vi "Sequencer Main.vi"() -> ()   [LabVIEW 2018] (continued)
                              # "Calculate Values"
                              n2034 = local read "Channel A"() -> (w4088:cluster{i32, dbl, dbl[]})
                              n2035 = local read "Channel B"() -> (w4085:cluster{i32, dbl, dbl[]})
                              n2036 = Unbundle(w4088) -> (w4093:dbl[])  [unwired: 2 out]
                              n2037 = Unbundle(w4085) -> (w4097:dbl[])  [unwired: 2 out]
                              n2038 = Array Size(array=w4093) -> (size(s)=w4099:i32)
                              n2039 = Array Size(array=w4097) -> (size(s)=w4096:i32)
                              n2040 = Subtract(x=w4099, y=w4095) -> (x-y=w4098:i32)
                              n2041 = Array Subset(array=w4093, index=w4095, length=w4098) -> (w4076:dbl[])
                              n2042 = Add(x=290, y="Correction") -> (x+y=w4077:i32)
                              "Pico Scope Correction" <- w4077
                              n2043 = Subtract(x=w4096, y=w4095) -> (x-y=w4094:i32)
                              n2044 = Array Subset(array=w4097, index=w4095, length=w4094) -> (w4090:dbl[])
                              n2045 = call "Wave Filter.vi"("Filter ON"=w4064, "Value"="F-Value", "Data In"=w4076) -> ("Data Out"=w4086:dbl[])  [unwired: 8 in]
                              n2046 = call "Wave Filter.vi"("Filter ON"=w4064, "Value"="F-Value", "Data In"=w4090) -> ("Data Out"=w4081:dbl[])  [unwired: 8 in]
                              n2047 = call "Convert to Dynamic Data"("Array"=w4086) -> ("Dynamic Data Type"=w4073:dynamicdata)  [unwired: 3 in]
                              n2048 = call "Convert to Dynamic Data2"("Array"=w4081) -> ("Dynamic Data Type"=w4072:dynamicdata)  [unwired: 3 in]
                              n2049 = Bundle(cluster=w4085, w4081) -> (w4084:cluster{i32, dbl, dbl[]})  [unwired: 2 in]
                              n2050 = call "Amplitude and Level Measurements2"("Signals"=w4072) -> ("Mean (DC)"=w4074:dynamicdata, "Negative Peak"=w4079:dynamicdata, "Positive Peak"=w4080:dynamicdata, "Peak to Peak"=w4070:dynamicdata)  [unwired: 10 in, 1 out]
                              n2051 = Bundle(cluster=w4088, w4086) -> (w4087:cluster{i32, dbl, dbl[]})  [unwired: 2 in]
                              n2052 = call "Amplitude and Level Measurements"("Signals"=w4073) -> ("Mean (DC)"=w4075:dynamicdata, "Negative Peak"=w4082:dynamicdata, "Positive Peak"=w4083:dynamicdata, "Peak to Peak"=w4067:dynamicdata)  [unwired: 10 in, 1 out]
                              n2053 = local write "Channel B"(w4084) -> ()
                              n2054 = Divide(x=w4067, y=2.0) -> (x/y=w4066:dynamicdata)
                              n2055 = Divide(x=w4070, y=2.0) -> (x/y=w4069:dynamicdata)
                              n2056 = local write "Channel A"(w4087) -> ()
                              n2057 = Subtract(1:w4075, 2:w4083) -> (0:w4109:dynamicdata)  [unwired: 1 in, 1 out]
                              n2058 = Add(1:w4075, 2:w4082) -> (0:w4108:dynamicdata)  [unwired: 1 in, 1 out]
                              n2059 = Subtract(1:w4074, 2:w4080) -> (0:w4105:dynamicdata)  [unwired: 1 in, 1 out]
                              n2060 = Add(1:w4074, 2:w4079) -> (0:w4104:dynamicdata)  [unwired: 1 in, 1 out]
                              n2061 = Multiply(x=w4066, y=w4077) -> (x*y=w4107:dynamicdata)
                              n2062 = Multiply(x=w4109, y=w4077) -> (x*y=w4103:dynamicdata)
                              n2063 = Multiply(x=w4108, y=w4077) -> (x*y=w4102:dynamicdata)
                              n2064 = local read "Measure Ch-A"() -> (w4113:T10)
                              n2065 = Multiply(x=w4069, y=w4077) -> (x*y=w4106:dynamicdata)
                              n2066 = Multiply(x=w4105, y=w4077) -> (x*y=w4101:dynamicdata)
                              n2067 = Multiply(x=w4104, y=w4077) -> (x*y=w4100:dynamicdata)
                              n2068 = Bundle By Name(cluster=w4113, "MAX Vpp"=w4103, "PickToPoick / 2"=w4107, "MIN Vpp"=w4102) -> (w4112:T10)
                              n2069 = local read "Measure Ch-B"() -> (w4110:T9)
                              n2070 = Bundle By Name(cluster=w4110, "MAX Vpp"=w4101, "PickToPick / 2"=w4106, "MIN Vpp"=w4100) -> (w4111:T9)
                              n2071 = local write "Measure Ch-B"(w4111) -> ()
                              n2072 = local write "Measure Ch-A"(w4112) -> ()
                            }
                            frame #2 {
                              # "GoTo Test-nmb"
                              # "ReTest Cyckles"
                              # "Select Channel & Set Retest Parametrs in FALSE Case"
                              n2073 = Index Array(array=w4131, index #1=0 ("index"), index #2=1 ("index"), index #3=2 ("index")) -> (element #1=w4135:string, element #2=w4136:string, element #3=w4137:string)
                              n2074 = global read "Global Variable.vi" "Retest Cnt"() -> (w4130:i16)
                              n2075 = local read "Debugging"() -> (w4128:bool)
                              n2076 = To Upper Case(1:w4135) -> (0:w4127:string)
                              n2077 = call "Convert from Dynamic Data"("Dynamic Data Type"=w4123) -> ("Scalar"=w4119:dbl)  [unwired: 3 in]
                              n2078 = call "Convert from Dynamic Data2"("Dynamic Data Type"=w4122) -> ("Scalar"=w4118:dbl)  [unwired: 3 in]
                              n2079 = call "Convert from Dynamic Data3"("Dynamic Data Type"=w4121) -> ("Scalar"=w4117:dbl)  [unwired: 3 in]
                              n2080 = call "Convert from Dynamic Data4"("Dynamic Data Type"=w4120) -> ("Scalar"=w4116:dbl)  [unwired: 3 in]
                              n2081 = Decimal String To Number(string=w4137) -> (number=w4124:i32)  [unwired: 2 in, 1 out]
                              n2082 = Decimal String To Number(string=w4136) -> (number=w4126:i32)  [unwired: 2 in, 1 out]
                              n2083 = Equal?(x=w4130, y=i16 0) -> (x = y?=w4125:bool)
                              n2084 = case shown="False" w4128 {
                                tunnel: w4127 -> [w4142 _]
                                tunnel: w4125 -> [w4139 _]
                                tunnel: w4124 -> [w4141 _]
                                tunnel: w4126 -> [w4140 _]
                                frame False {
                                n2085 = case shown="\"FALSE\"" w4142 {
                                tunnel: w4139 -> [_ w4146]
                                tunnel: w4141 -> [_ w4143]
                                tunnel: w4140 -> [_ w4144]
                                frame "Idle", Default {
                                }
                                frame "FALSE" {
                                n2086 = global write "Global Variable.vi" "Retest Step Nmb"(w4144) -> ()
                                n2087 = global write "Global Variable.vi" "Retest Nmb"(w4143) -> ()
                                n2088 = case shown="True" w4146 {
                                tunnel: w4143 -> [_ w4150]
                                tunnel: w4144 -> [_ _]
                                frame False {
                                n2089 = global read "Global Variable.vi" "Retest Cnt"() -> (w4148:i16)
                                n2090 = Decrement(x=w4148) -> (x-1=w4147:i16)
                                n2091 = global write "Global Variable.vi" "Retest Cnt"(w4147) -> ()
                                }
                                frame True {
                                # "if(Retest-OFF & Cnt=0)"
                                n2092 = Decrement(x=w4150) -> (x-1=w4149:i32)
                                n2093 = global write "Global Variable.vi" "Retest Cnt"(w4149) -> ()
                                }
                                }
                                n2094 = global write "Global Variable.vi" "Retest ON"(TRUE ("Retest ON")) -> ()
                                }
                                }
                                }
                                frame True {
                                }
                              }
                              n2095 = case shown="\"A\", Default" w4138 {
                                tunnel: [w4152 w4154] -> w4115
                                tunnel: w4119 -> [w4152 _]
                                tunnel: w4118 -> [w4151 _]
                                tunnel: [w4151 w4153] -> w4114
                                tunnel: w4117 -> [_ w4154]
                                tunnel: w4116 -> [_ w4153]
                                frame "A", Default {
                                }
                                frame "B" {
                                }
                              }
                            }
                            frame #3 {
                              # "Negative MIN"
                              # "Positive MAX"
                              n2096 = Multiply(x="Delay", y=u32 1000 ("milliseconds to wait")) -> (x*y=w4157:u32)
                              n2097 = Wait (ms)(milliseconds to wait=w4157) -> ()  [unwired: 1 out]
                            }
                          }
                          n2098 = in-place {
                            in-place-border: w3995 -> [w4019]
                            in-place-border: w3993 -> [w4018]
                            in-place-border: w3996 -> [w4025]
                            in-place-border: w3997 -> [w4024]
                            in-place-border: [w4026] -> w3991
                            in-place-border: [w4017] -> w3990
                            # "Step Result Msg"
                            # "Step TEST Result"
                            n2099 = in-place {
                              in-place-border: w4025 -> [w4030]
                              in-place-border: w4024 -> [w4027]
                              in-place-border: [w4030] -> w4023
                              in-place-border: [w4029] -> w4021
                              in-place-border: [w4028] -> w4020
                              in-place-border: [w4027] -> w4022
                              n2100 = Multiply(x=w4027, y=-1.0) -> (x*y=w4028:dbl)
                              n2101 = Multiply(x=w4030, y=-1.0) -> (x*y=w4029:dbl)
                            }
                            n2102 = In Range and Coerce(upper limit=w4023, x=w4019, lower limit=w4022) -> (In Range?=w4015:bool)  [unwired: 1 out]
                            n2103 = In Range and Coerce(upper limit=w4020, x=w4018, lower limit=w4021) -> (In Range?=w4014:bool)  [unwired: 1 out]
                            n2104 = And(x=w4015, y=w4014) -> (x .and. y?=w4013:bool)
                            n2105 = case shown="False" w4013 {
                              tunnel: [enum16{"Idle", "PASS", "FALSE"}."FALSE" ("Step Test Result") enum16{"Idle", "PASS", "FALSE"}."PASS" ("Step Test Result")] -> w4026
                              frame False {
                              }
                              frame True {
                              }
                            }
                            n2106 = Format Into String(format string="Max: %.1fVAC :: Min: %.1fVAC", w4019, w4018) -> (resulting string=w4017:string)  [unwired: 2 in, 1 out]
                          }
                        }
                        frame 56 {
                          # "Read Peack To Peak / 2"
                          # "Lover Lim"
                          # "Upper Lim"
                          # "PicoScope"
                          # "PicoScope Case"
                          n2107 = Unbundle By Name(w4178) -> ("Parameters"=w4172:string, "Test Values.Upper Limit"=w4176:dbl, "Test Values.Lower Limit"=w4175:dbl, "Test Values.Numeric Value"=w4177:dbl)
                          n2108 = property on="Tab Control Msg" class="TabCtl (strict)"("Value"=T21."Scope" ("Tab Control Msg")) -> (error out=w4174:errorcluster)  [unwired: 2 in, 1 out]
                          n2109 = flat-sequence {
                            tunnel: w4177 -> [w4205]
                            tunnel: w4176 -> [w4198]
                            tunnel: w4175 -> [w4197]
                            tunnel: w4174 -> [_]
                            tunnel: [w4198] -> w4164
                            tunnel: [w4197] -> w4165
                            tunnel: w4172 -> [w4196]
                            tunnel: [w4194] -> w4169
                            tunnel: [w4190] -> w4166
                            tunnel: [w4224] -> w4171
                            tunnel: [w4223] -> w4170
                            tunnel: w4169 -> [w4249]
                            tunnel: [w4249] -> w4168
                            tunnel: [w4248] -> w4167
                            tunnel: w4166 -> [w4248]
                            tunnel: w4171 -> [w4273]
                            tunnel: w4170 -> [w4272]
                            tunnel: w4168 -> [w4288]
                            tunnel: w4167 -> [w4281]
                            tunnel: [w4271] -> w4162
                            tunnel: [w4304] -> w4163
                            tunnel: w4162 -> [w4304]
                            frame #0 {
                              n2110 = while {
                                shift-right: [w4216] -> _
                                shift-left: w4196 -> [w4217]
                                tunnel: [w4213] -> w4195 mode=indexing
                                stop <- w4215 stop-if-true
                                # "Get Array of Parametrs"
                                n2111 = Match Pattern(string=w4217, regular expression=">") -> (before substring=w4213:string, after substring=w4216:string, offset past match=w4214:i32)  [unwired: 1 in, 1 out]
                                n2112 = Less Than 0?(x=w4214) -> (x < 0?=w4215:bool)
                              }
                              n2113 = Multiply(x=w4197, y=-0.2) -> (x*y=w4200:dbl)
                              n2114 = Bundle("Lower Limit"=w4197, "Upper Limit"=w4198, "Numeric Value"=w4205) -> (w4206:T36)  [unwired: 1 in]
                              n2115 = Multiply(x=w4198, y=0.2) -> (x*y=w4202:dbl)
                              n2116 = Add(x=w4200, y=w4197) -> (x+y=w4199:dbl)
                              n2117 = property on="Limits" class="Slide (strict)"("Value"=w4206) -> ()  [unwired: 2 in, 2 out]
                              n2118 = Add(x=w4202, y=w4198) -> (x+y=w4201:dbl)
                              n2119 = property on="Limits" class="Slide (strict)"("Scale.Maximum"=w4201, "Scale.Minimum"=w4199) -> ()  [unwired: 2 in, 2 out]
                              n2120 = Index Array(array=w4195, index #1=0 ("index"), index #2=1 ("index")) -> (element #1=w4194:string, element #2=w4191:string)
                              n2121 = while {
                                shift-right: [w4210] -> _
                                shift-left: w4191 -> [w4211]
                                tunnel: [w4207] -> w4190 mode=indexing
                                stop <- w4209 stop-if-true
                                # "Get Array of Sub Parametrs"
                                n2122 = Match Pattern(string=w4211, regular expression=":") -> (before substring=w4207:string, after substring=w4210:string, offset past match=w4208:i32)  [unwired: 1 in, 1 out]
                                n2123 = Less Than 0?(x=w4208) -> (x < 0?=w4209:bool)
                              }
                            }
                            frame #1 {
                              w4219 = TRUE
                              w4252 = 100 ("index")
                              # "700"
                              # "Devider compensite"
                              # "remove first\nxx element (noise)"
                              # "Ch-B Peack To Peack / 2"
                              # "Ch-A Peack To Peack / 2"
                              # "Res Devider Compens\n100K / 10K"
                              # "Calculate Values"
                              n2124 = local read "Correction"() -> (w4222:i32)
                              n2125 = local read "Channel A"() -> (w4246:cluster{i32, dbl, dbl[]})
                              n2126 = local read "Channel B"() -> (w4243:cluster{i32, dbl, dbl[]})
                              n2127 = Unbundle(w4246) -> (w4250:dbl[])  [unwired: 2 out]
                              n2128 = Unbundle(w4243) -> (w4254:dbl[])  [unwired: 2 out]
                              n2129 = local read "F-Value"() -> (w4220:dbl)
                              n2130 = Array Size(array=w4250) -> (size(s)=w4256:i32)
                              n2131 = Array Size(array=w4254) -> (size(s)=w4253:i32)
                              n2132 = Subtract(x=w4256, y=w4252) -> (x-y=w4255:i32)
                              n2133 = Array Subset(array=w4250, index=w4252, length=w4255) -> (w4235:dbl[])
                              n2134 = Add(x=290, y=w4222) -> (x+y=w4221:i32)
                              n2135 = Subtract(x=w4253, y=w4252) -> (x-y=w4251:i32)
                              n2136 = Array Subset(array=w4254, index=w4252, length=w4251) -> (w4247:dbl[])
                              n2137 = call "Wave Filter.vi"("Filter ON"=w4219, "Value"=w4220, "Data In"=w4235) -> ("Data Out"=w4244:dbl[])  [unwired: 8 in]
                              n2138 = call "Wave Filter.vi"("Filter ON"=w4219, "Value"=w4220, "Data In"=w4247) -> ("Data Out"=w4239:dbl[])  [unwired: 8 in]
                              n2139 = local write "Pico Scope Correction"(w4221) -> ()
                              n2140 = call "Convert to Dynamic Data4"("Array"=w4244) -> ("Dynamic Data Type"=w4232:dynamicdata)  [unwired: 3 in]
                              n2141 = call "Convert to Dynamic Data3"("Array"=w4239) -> ("Dynamic Data Type"=w4231:dynamicdata)  [unwired: 3 in]
                              n2142 = Bundle(cluster=w4243, w4239) -> (w4242:cluster{i32, dbl, dbl[]})  [unwired: 2 in]
                              n2143 = call "Amplitude and Level Measurements4"("Signals"=w4231) -> ("Mean (DC)"=w4233:dynamicdata, "Negative Peak"=w4237:dynamicdata, "Positive Peak"=w4238:dynamicdata, "Peak to Peak"=w4230:dynamicdata)  [unwired: 10 in, 1 out]
                              n2144 = Bundle(cluster=w4246, w4244) -> (w4245:cluster{i32, dbl, dbl[]})  [unwired: 2 in]
                              n2145 = call "Amplitude and Level Measurements3"("Signals"=w4232) -> ("Mean (DC)"=w4234:dynamicdata, "Negative Peak"=w4240:dynamicdata, "Positive Peak"=w4241:dynamicdata, "Peak to Peak"=w4227:dynamicdata)  [unwired: 10 in, 1 out]
                              n2146 = local write "Channel B"(w4242) -> ()
                              n2147 = Divide(x=w4227, y=2.0) -> (x/y=w4226:dynamicdata)
                              n2148 = Divide(x=w4230, y=2.0) -> (x/y=w4229:dynamicdata)
                              n2149 = local write "Channel A"(w4245) -> ()
                              n2150 = Subtract(1:w4234, 2:w4241) -> (0:w4264:dynamicdata)  [unwired: 1 in, 1 out]
                              n2151 = Add(1:w4234, 2:w4240) -> (0:w4263:dynamicdata)  [unwired: 1 in, 1 out]
                              n2152 = Subtract(1:w4233, 2:w4238) -> (0:w4262:dynamicdata)  [unwired: 1 in, 1 out]
                              n2153 = Add(1:w4233, 2:w4237) -> (0:w4261:dynamicdata)  [unwired: 1 in, 1 out]
                              n2154 = Multiply(x=w4226, y=w4221) -> (x*y=w4224:dynamicdata)
                              n2155 = Multiply(x=w4264, y=w4221) -> (x*y=w4260:dynamicdata)
                              n2156 = Multiply(x=w4263, y=w4221) -> (x*y=w4259:dynamicdata)
                              n2157 = local read "Measure Ch-A"() -> (w4268:T10)
                              n2158 = Multiply(x=w4229, y=w4221) -> (x*y=w4223:dynamicdata)
                              n2159 = Multiply(x=w4262, y=w4221) -> (x*y=w4258:dynamicdata)
                              n2160 = Multiply(x=w4261, y=w4221) -> (x*y=w4257:dynamicdata)
                              n2161 = Bundle By Name(cluster=w4268, "MAX Vpp"=w4260, "PickToPoick / 2"=w4224, "MIN Vpp"=w4259) -> (w4267:T10)
                              n2162 = local read "Measure Ch-B"() -> (w4265:T9)
                              n2163 = Bundle By Name(cluster=w4265, "MAX Vpp"=w4258, "PickToPick / 2"=w4223, "MIN Vpp"=w4257) -> (w4266:T9)
                              n2164 = local write "Measure Ch-B"(w4266) -> ()
                              n2165 = local write "Measure Ch-A"(w4267) -> ()
                            }
                            frame #2 {
                              # "GoTo Test-nmb"
                              # "ReTest Cyckles"
                              # "Select Channel & Set Retest Parametrs in FALSE Case"
                              n2166 = Index Array(array=w4281, index #1=0 ("index"), index #2=1 ("index"), index #3=2 ("index")) -> (element #1=w4285:string, element #2=w4286:string, element #3=w4287:string)
                              n2167 = global read "Global Variable.vi" "Retest Cnt"() -> (w4280:i16)
                              n2168 = local read "Debugging"() -> (w4278:bool)
                              n2169 = To Upper Case(1:w4285) -> (0:w4277:string)
                              n2170 = call "Convert from Dynamic Data8"("Dynamic Data Type"=w4273) -> ("Scalar"=w4269:dbl)  [unwired: 3 in]
                              n2171 = call "Convert from Dynamic Data6"("Dynamic Data Type"=w4272) -> ("Scalar"=w4270:dbl)  [unwired: 3 in]
                              n2172 = Decimal String To Number(string=w4287) -> (number=w4274:i32)  [unwired: 2 in, 1 out]
                              n2173 = Decimal String To Number(string=w4286) -> (number=w4276:i32)  [unwired: 2 in, 1 out]
                              n2174 = Equal?(x=w4280, y=i16 0) -> (x = y?=w4275:bool)
                              n2175 = case shown="False" w4278 {
                                tunnel: w4277 -> [w4292 _]
                                tunnel: w4275 -> [w4289 _]
                                tunnel: w4274 -> [w4291 _]
                                tunnel: w4276 -> [w4290 _]
                                frame False {
                                n2176 = case shown="\"FALSE\"" w4292 {
                                tunnel: w4289 -> [_ w4296]
                                tunnel: w4291 -> [_ w4293]
                                tunnel: w4290 -> [_ w4294]
                                frame "Idle", Default {
                                }
                                frame "FALSE" {
                                n2177 = global write "Global Variable.vi" "Retest Step Nmb"(w4294) -> ()
                                n2178 = global write "Global Variable.vi" "Retest Nmb"(w4293) -> ()
                                n2179 = case shown="True" w4296 {
                                tunnel: w4293 -> [_ w4300]
                                tunnel: w4294 -> [_ _]
                                frame False {
                                n2180 = global read "Global Variable.vi" "Retest Cnt"() -> (w4298:i16)
                                n2181 = Decrement(x=w4298) -> (x-1=w4297:i16)
                                n2182 = global write "Global Variable.vi" "Retest Cnt"(w4297) -> ()
                                }
                                frame True {
                                # "if(Retest-OFF & Cnt=0)"
                                n2183 = Decrement(x=w4300) -> (x-1=w4299:i32)
                                n2184 = global write "Global Variable.vi" "Retest Cnt"(w4299) -> ()
                                }
                                }
                                n2185 = global write "Global Variable.vi" "Retest ON"(TRUE ("Retest ON")) -> ()
                                }
                                }
                                }
                                frame True {
                                }
                              }
                              n2186 = case shown="\"A\", Default" w4288 {
                                tunnel: [w4301 w4302] -> w4271
                                tunnel: w4270 -> [_ w4302]
                                tunnel: w4269 -> [w4301 _]
                                frame "A", Default {
                                }
                                frame "B" {
                                }
                              }
                            }
                            frame #3 {
                              n2187 = local read "Delay"() -> (w4303:u16)
                              n2188 = Multiply(x=w4303, y=u32 1000 ("milliseconds to wait")) -> (x*y=w4305:u32)
                              n2189 = Wait (ms)(milliseconds to wait=w4305) -> ()  [unwired: 1 out]
                            }
                          }
                          n2190 = in-place {
                            in-place-border: w4163 -> [w4186]
                            in-place-border: w4164 -> [w4180]
                            in-place-border: w4165 -> [w4179]
                            in-place-border: [w4187] -> w4161
                            in-place-border: [w4185] -> w4160
                            # "Step Result Msg"
                            # "Step TEST Result"
                            n2191 = In Range and Coerce(upper limit=w4180, x=w4186, lower limit=w4179) -> (In Range?=w4183:bool)  [unwired: 1 out]
                            n2192 = And(x=w4183, y=TRUE) -> (x .and. y?=w4182:bool)
                            n2193 = case shown="False" w4182 {
                              tunnel: [enum16{"Idle", "PASS", "FALSE"}."FALSE" ("Step Test Result") enum16{"Idle", "PASS", "FALSE"}."PASS" ("Step Test Result")] -> w4187
                              frame False {
                              }
                              frame True {
                              }
                            }
                            n2194 = Format Into String(format string="%.1f (V)", w4186) -> (resulting string=w4185:string)  [unwired: 2 in, 1 out]
                          }
                        }
                        frame 53 {
                          # "Read Only POSITIVE or NEGATIVE Values"
                          # "Read Arrays Of DATA"
                          # "Lover Lim"
                          # "Upper Lim"
                          # "PicoScope Case\nPositive / Negative"
                          # "PicoScope Case"
                          n2195 = Unbundle By Name(w4330) -> ("Parameters"=w4324:string, "Test Values.Upper Limit"=w4328:dbl, "Test Values.Lower Limit"=w4327:dbl, "Test Values.Numeric Value"=w4329:dbl)
                          n2196 = property on="Tab Control Msg" class="TabCtl (strict)"("Value"=T21."Scope" ("Tab Control Msg")) -> (error out=w4326:errorcluster)  [unwired: 2 in, 1 out]
                          n2197 = flat-sequence {
                            tunnel: w4329 -> [w4362]
                            tunnel: w4328 -> [w4355]
                            tunnel: w4327 -> [w4354]
                            tunnel: w4326 -> [_]
                            tunnel: [w4355] -> w4314
                            tunnel: [w4354] -> w4315
                            tunnel: w4324 -> [w4353]
                            tunnel: [w4351] -> w4319
                            tunnel: [w4348] -> w4316
                            tunnel: [w4345] -> w4308
                            tunnel: [w4393] -> w4323
                            tunnel: [w4392] -> w4322
                            tunnel: [w4391] -> w4321
                            tunnel: [w4390] -> w4320
                            tunnel: w4319 -> [w4379]
                            tunnel: [w4379] -> w4318
                            tunnel: [w4378] -> w4317
                            tunnel: w4316 -> [w4378]
                            tunnel: [w4376] -> w4309
                            tunnel: w4308 -> [w4376]
                            tunnel: [w4433] -> w4313
                            tunnel: [w4435] -> w4312
                            tunnel: w4323 -> [w4434]
                            tunnel: w4322 -> [w4432]
                            tunnel: w4321 -> [w4431]
                            tunnel: w4320 -> [w4430]
                            tunnel: w4318 -> [w4429]
                            tunnel: w4317 -> [w4422]
                            tunnel: w4309 -> [w4414]
                            tunnel: [w4413] -> w4307
                            frame #0 {
                              n2198 = while {
                                shift-right: [w4373] -> _
                                shift-left: w4353 -> [w4374]
                                tunnel: [w4370] -> w4352 mode=indexing
                                stop <- w4372 stop-if-true
                                # "Get Array of Parametrs"
                                n2199 = Match Pattern(string=w4374, regular expression=">") -> (before substring=w4370:string, after substring=w4373:string, offset past match=w4371:i32)  [unwired: 1 in, 1 out]
                                n2200 = Less Than 0?(x=w4371) -> (x < 0?=w4372:bool)
                              }
                              n2201 = Multiply(x=w4354, y=-0.2) -> (x*y=w4357:dbl)
                              n2202 = Bundle("Lower Limit"=w4354, "Upper Limit"=w4355, "Numeric Value"=w4362) -> (w4363:T36)  [unwired: 1 in]
                              n2203 = Multiply(x=w4355, y=0.2) -> (x*y=w4359:dbl)
                              n2204 = Add(x=w4357, y=w4354) -> (x+y=w4356:dbl)
                              n2205 = property on="Limits" class="Slide (strict)"("Value"=w4363) -> ()  [unwired: 2 in, 2 out]
                              n2206 = Add(x=w4359, y=w4355) -> (x+y=w4358:dbl)
                              n2207 = property on="Limits" class="Slide (strict)"("Scale.Maximum"=w4358, "Scale.Minimum"=w4356) -> ()  [unwired: 2 in, 2 out]
                              n2208 = Index Array(array=w4352, index #1=0 ("index"), index #2=1 ("index"), index #3=2 ("index")) -> (element #1=w4351:string, element #2=w4345:string, element #3=w4346:string)
                              n2209 = while {
                                shift-right: [w4367] -> _
                                shift-left: w4346 -> [w4368]
                                tunnel: [w4364] -> w4348 mode=indexing
                                stop <- w4366 stop-if-true
                                # "Get Array of Sub Parametrs"
                                n2210 = Match Pattern(string=w4368, regular expression=":") -> (before substring=w4364:string, after substring=w4367:string, offset past match=w4365:i32)  [unwired: 1 in, 1 out]
                                n2211 = Less Than 0?(x=w4365) -> (x < 0?=w4366:bool)
                              }
                            }
                            frame #1 {
                              w4383 = 700 ("index")
                              w4377 = 290.0
                              # "302"
                              # "Devider compensite"
                              # "remove first\nxx element (noise)"
                              # "Ch-B Negative Vmin"
                              # "Ch-B Positive Vmax"
                              # "Ch-A Negative Vmin"
                              # "Ch-A Positive Vmax"
                              # "Res Devider Compens\n100K / 10K"
                              # "Calculate Values"
                              n2212 = local read "Channel A"() -> (w4412:cluster{i32, dbl, dbl[]})
                              n2213 = local read "Channel B"() -> (w4407:cluster{i32, dbl, dbl[]})
                              n2214 = Unbundle(w4412) -> (w4380:dbl[])  [unwired: 2 out]
                              n2215 = Unbundle(w4407) -> (w4385:dbl[])  [unwired: 2 out]
                              n2216 = Array Size(array=w4380) -> (size(s)=w4388:i32)
                              n2217 = Array Size(array=w4385) -> (size(s)=w4384:i32)
                              n2218 = Subtract(x=w4388, y=w4383) -> (x-y=w4387:i32)
                              n2219 = Array Subset(array=w4380, index=w4383, length=w4387) -> (w4389:dbl[])
                              n2220 = Subtract(x=w4384, y=w4383) -> (x-y=w4382:i32)
                              n2221 = Array Subset(array=w4385, index=w4383, length=w4382) -> (w4386:dbl[])
                              n2222 = call-poly <vilib>:"Basic Averaged DC-RMS.vi"("signal in"=w4389) -> ("RMS value"=w4401:dbl, "DC value"=w4381:dbl)  [unwired: 7 in, 2 out]
                              n2223 = Array Max & Min(array=w4389) -> (max value=w4409:dbl, min value=w4408:dbl)  [unwired: 2 out]
                              n2224 = call-poly <vilib>:"Basic Averaged DC-RMS.vi"("signal in"=w4386) -> ("RMS value"=w4397:dbl, "DC value"=w4406:dbl)  [unwired: 7 in, 2 out]
                              n2225 = Array Max & Min(array=w4386) -> (max value=w4404:dbl, min value=w4405:dbl)  [unwired: 2 out]
                              n2226 = Subtract(x=w4409, y=w4381) -> (x-y=w4400:dbl)
                              n2227 = Add(x=w4408, y=w4381) -> (x+y=w4399:dbl)
                              n2228 = Subtract(x=w4404, y=w4406) -> (x-y=w4395:dbl)
                              n2229 = Add(x=w4405, y=w4406) -> (x+y=w4394:dbl)
                              n2230 = Multiply(x=w4401, y=w4377) -> (x*y=w4398:dbl)
                              n2231 = Multiply(x=w4400, y=w4377) -> (x*y=w4393:dbl)
                              n2232 = Multiply(x=w4399, y=w4377) -> (x*y=w4392:dbl)
                              n2233 = Multiply(x=w4397, y=w4377) -> (x*y=w4396:dbl)
                              n2234 = Multiply(x=w4395, y=w4377) -> (x*y=w4391:dbl)
                              n2235 = Multiply(x=w4394, y=w4377) -> (x*y=w4390:dbl)
                              n2236 = local read "Measure Ch-A"() -> (w4411:T10)
                              n2237 = Bundle By Name(cluster=w4411, "MAX Vpp"=w4393, "PickToPoick / 2"=w4398, "MIN Vpp"=w4392) -> (w4410:T10)
                              n2238 = local read "Measure Ch-B"() -> (w4402:T9)
                              n2239 = local write "Measure Ch-A"(w4410) -> ()
                              n2240 = Bundle By Name(cluster=w4402, "MAX Vpp"=w4391, "PickToPick / 2"=w4396, "MIN Vpp"=w4390) -> (w4403:T9)
                              n2241 = local write "Measure Ch-B"(w4403) -> ()
                            }
                            frame #2 {
                              # "Negative"
                              # "Positive"
                              # "GoTo Test-nmb"
                              # "ReTest Cyckles"
                              # "Select Channel & Set Retest Parametrs in FALSE Case"
                              n2242 = Index Array(array=w4422, index #1=0 ("index"), index #2=1 ("index"), index #3=2 ("index")) -> (element #1=w4426:string, element #2=w4427:string, element #3=w4428:string)
                              n2243 = global read "Global Variable.vi" "Retest Cnt"() -> (w4421:i16)
                              n2244 = local read "Debugging"() -> (w4419:bool)
                              n2245 = To Upper Case(1:w4426) -> (0:w4418:string)
                              n2246 = Decimal String To Number(string=w4428) -> (number=w4415:i32)  [unwired: 2 in, 1 out]
                              n2247 = Decimal String To Number(string=w4427) -> (number=w4417:i32)  [unwired: 2 in, 1 out]
                              n2248 = Equal?(x=w4421, y=i16 0) -> (x = y?=w4416:bool)
                              n2249 = case shown="False" w4419 {
                                tunnel: w4418 -> [w4439 _]
                                tunnel: w4416 -> [w4436 _]
                                tunnel: w4415 -> [w4438 _]
                                tunnel: w4417 -> [w4437 _]
                                frame False {
                                n2250 = case shown="\"FALSE\"" w4439 {
                                tunnel: w4436 -> [_ w4443]
                                tunnel: w4438 -> [_ w4440]
                                tunnel: w4437 -> [_ w4441]
                                frame "Idle", Default {
                                }
                                frame "FALSE" {
                                n2251 = global write "Global Variable.vi" "Retest Step Nmb"(w4441) -> ()
                                n2252 = global write "Global Variable.vi" "Retest Nmb"(w4440) -> ()
                                n2253 = case shown="True" w4443 {
                                tunnel: w4440 -> [_ w4447]
                                tunnel: w4441 -> [_ _]
                                frame False {
                                n2254 = global read "Global Variable.vi" "Retest Cnt"() -> (w4445:i16)
                                n2255 = Decrement(x=w4445) -> (x-1=w4444:i16)
                                n2256 = global write "Global Variable.vi" "Retest Cnt"(w4444) -> ()
                                }
                                frame True {
                                # "if(Retest-OFF & Cnt=0)"
                                n2257 = Decrement(x=w4447) -> (x-1=w4446:i32)
                                n2258 = global write "Global Variable.vi" "Retest Cnt"(w4446) -> ()
                                }
                                }
                                n2259 = global write "Global Variable.vi" "Retest ON"(TRUE ("Retest ON")) -> ()
                                }
                                }
                                }
                                frame True {
                                }
                              }
                              n2260 = case shown="\"A\", Default" w4429 {
                                tunnel: [w4449 w4451] -> w4435
                                tunnel: w4434 -> [w4449 _]
                                tunnel: [w4448 w4450] -> w4433
                                tunnel: w4432 -> [w4448 _]
                                tunnel: w4431 -> [_ w4451]
                                tunnel: w4430 -> [_ w4450]
                                frame "A", Default {
                                }
                                frame "B" {
                                }
                              }
                              n2261 = To Lower Case(string=w4414) -> (all lower case string=w4413:string)
                            }
                          }
                          n2262 = in-place {
                            in-place-border: w4312 -> [w4333]
                            in-place-border: w4313 -> [w4332]
                            in-place-border: w4314 -> [w4336]
                            in-place-border: w4315 -> [w4335]
                            in-place-border: [w4340] -> w4311
                            in-place-border: [w4339] -> w4310
                            in-place-border: w4307 -> [w4334]
                            # "Upper Limit Check"
                            # "Step Result Msg"
                            # "Step TEST Result"
                            n2263 = case shown="\"positive\", Default" w4334 {
                              tunnel: w4333 -> [_ w4342]
                              tunnel: w4332 -> [w4341 _]
                              tunnel: [w4341 w4342] -> w4331
                              frame "negative" {
                              }
                              frame "positive", Default {
                              }
                            }
                            n2264 = Format Into String(format string="%.1f (VAC )", w4331) -> (resulting string=w4339:string)  [unwired: 2 in, 1 out]
                            n2265 = In Range and Coerce(upper limit=w4336, x=w4331, lower limit=w4335) -> (In Range?=w4337:bool)  [unwired: 1 out]
                            n2266 = case shown="False" w4337 {
                              tunnel: [enum16{"Idle", "PASS", "FALSE"}."FALSE" ("Step Test Result") enum16{"Idle", "PASS", "FALSE"}."PASS" ("Step Test Result")] -> w4340
                              frame False {
                              }
                              frame True {
                              }
                            }
                          }
                        }
                        frame 54 {
                          # "PicoScope\n     Case\nLower Limit"
                          # "Read Arrays Of DATA"
                          # "Lover Lim"
                          # "Upper Lim"
                          # "PicoScope Case"
                          n2267 = Unbundle By Name(w4472) -> ("Parameters"=w4464:string, "Test Values.Upper Limit"=w4470:dbl, "Test Values.Lower Limit"=w4469:dbl, "Test Values.Numeric Value"=w4471:dbl)
                          n2268 = property on="Tab Control Msg" class="TabCtl (strict)"("Value"=T21."Scope" ("Tab Control Msg")) -> (error out=w4468:errorcluster)  [unwired: 2 in, 1 out]
                          n2269 = flat-sequence {
                            tunnel: w4471 -> [w4497]
                            tunnel: w4470 -> [w4490]
                            tunnel: w4469 -> [w4489]
                            tunnel: w4468 -> [_]
                            tunnel: [w4490] -> w4454
                            tunnel: [w4489] -> w4455
                            tunnel: w4464 -> [w4488]
                            tunnel: [w4486] -> w4459
                            tunnel: [w4482] -> w4456
                            tunnel: [w4527] -> w4463
                            tunnel: [w4526] -> w4462
                            tunnel: [w4525] -> w4461
                            tunnel: [w4524] -> w4460
                            tunnel: w4459 -> [w4513]
                            tunnel: [w4513] -> w4458
                            tunnel: [w4512] -> w4457
                            tunnel: w4456 -> [w4512]
                            tunnel: [w4565] -> w4453
                            tunnel: [w4567] -> w4452
                            tunnel: w4463 -> [w4566]
                            tunnel: w4462 -> [w4564]
                            tunnel: w4461 -> [w4563]
                            tunnel: w4460 -> [w4562]
                            tunnel: w4458 -> [w4561]
                            tunnel: w4457 -> [w4554]
                            frame #0 {
                              n2270 = while {
                                shift-right: [w4508] -> _
                                shift-left: w4488 -> [w4509]
                                tunnel: [w4505] -> w4487 mode=indexing
                                stop <- w4507 stop-if-true
                                # "Get Array of Parametrs"
                                n2271 = Match Pattern(string=w4509, regular expression=">") -> (before substring=w4505:string, after substring=w4508:string, offset past match=w4506:i32)  [unwired: 1 in, 1 out]
                                n2272 = Less Than 0?(x=w4506) -> (x < 0?=w4507:bool)
                              }
                              n2273 = Multiply(x=w4489, y=-0.2) -> (x*y=w4492:dbl)
                              n2274 = Bundle("Lower Limit"=w4489, "Upper Limit"=w4490, "Numeric Value"=w4497) -> (w4498:T36)  [unwired: 1 in]
                              n2275 = Multiply(x=w4490, y=0.2) -> (x*y=w4494:dbl)
                              n2276 = Add(x=w4492, y=w4489) -> (x+y=w4491:dbl)
                              n2277 = property on="Limits" class="Slide (strict)"("Value"=w4498) -> ()  [unwired: 2 in, 2 out]
                              n2278 = Add(x=w4494, y=w4490) -> (x+y=w4493:dbl)
                              n2279 = property on="Limits" class="Slide (strict)"("Scale.Maximum"=w4493, "Scale.Minimum"=w4491) -> ()  [unwired: 2 in, 2 out]
                              n2280 = Index Array(array=w4487, index #1=0 ("index"), index #2=1 ("index")) -> (element #1=w4486:string, element #2=w4483:string)
                              n2281 = while {
                                shift-right: [w4502] -> _
                                shift-left: w4483 -> [w4503]
                                tunnel: [w4499] -> w4482 mode=indexing
                                stop <- w4501 stop-if-true
                                # "Get Array of Sub Parametrs"
                                n2282 = Match Pattern(string=w4503, regular expression=":") -> (before substring=w4499:string, after substring=w4502:string, offset past match=w4500:i32)  [unwired: 1 in, 1 out]
                                n2283 = Less Than 0?(x=w4500) -> (x < 0?=w4501:bool)
                              }
                            }
                            frame #1 {
                              w4517 = 700 ("index")
                              w4511 = 290.0
                              # "302"
                              # "Devider compensite"
                              # "remove first\nxx element (noise)"
                              # "Ch-B Negative Vmin"
                              # "Ch-B Positive Vmax"
                              # "Ch-A Negative Vmin"
                              # "Ch-A Positive Vmax"
                              # "Res Devider Compens\n100K / 10K"
                              # "Calculate Values"
                              n2284 = local read "Channel A"() -> (w4546:cluster{i32, dbl, dbl[]})
                              n2285 = local read "Channel B"() -> (w4541:cluster{i32, dbl, dbl[]})
                              n2286 = Unbundle(w4546) -> (w4514:dbl[])  [unwired: 2 out]
                              n2287 = Unbundle(w4541) -> (w4519:dbl[])  [unwired: 2 out]
                              n2288 = Array Size(array=w4514) -> (size(s)=w4522:i32)
                              n2289 = Array Size(array=w4519) -> (size(s)=w4518:i32)
                              n2290 = Subtract(x=w4522, y=w4517) -> (x-y=w4521:i32)
                              n2291 = Array Subset(array=w4514, index=w4517, length=w4521) -> (w4523:dbl[])
                              n2292 = Subtract(x=w4518, y=w4517) -> (x-y=w4516:i32)
                              n2293 = Array Subset(array=w4519, index=w4517, length=w4516) -> (w4520:dbl[])
                              n2294 = call-poly <vilib>:"Basic Averaged DC-RMS.vi"("signal in"=w4523) -> ("RMS value"=w4535:dbl, "DC value"=w4515:dbl)  [unwired: 7 in, 2 out]
                              n2295 = Array Max & Min(array=w4523) -> (max value=w4543:dbl, min value=w4542:dbl)  [unwired: 2 out]
                              n2296 = call-poly <vilib>:"Basic Averaged DC-RMS.vi"("signal in"=w4520) -> ("RMS value"=w4531:dbl, "DC value"=w4540:dbl)  [unwired: 7 in, 2 out]
                              n2297 = Array Max & Min(array=w4520) -> (max value=w4538:dbl, min value=w4539:dbl)  [unwired: 2 out]
                              n2298 = Subtract(x=w4543, y=w4515) -> (x-y=w4534:dbl)
                              n2299 = Add(x=w4542, y=w4515) -> (x+y=w4533:dbl)
                              n2300 = Subtract(x=w4538, y=w4540) -> (x-y=w4529:dbl)
                              n2301 = Add(x=w4539, y=w4540) -> (x+y=w4528:dbl)
                              n2302 = Multiply(x=w4535, y=w4511) -> (x*y=w4532:dbl)
                              n2303 = Multiply(x=w4534, y=w4511) -> (x*y=w4527:dbl)
                              n2304 = Multiply(x=w4533, y=w4511) -> (x*y=w4526:dbl)
                              n2305 = Multiply(x=w4531, y=w4511) -> (x*y=w4530:dbl)
                              n2306 = Multiply(x=w4529, y=w4511) -> (x*y=w4525:dbl)
                              n2307 = Multiply(x=w4528, y=w4511) -> (x*y=w4524:dbl)
                              n2308 = local read "Measure Ch-A"() -> (w4545:T10)
                              n2309 = Bundle By Name(cluster=w4545, "MAX Vpp"=w4527, "PickToPoick / 2"=w4532, "MIN Vpp"=w4526) -> (w4544:T10)
                              n2310 = local read "Measure Ch-B"() -> (w4536:T9)
                              n2311 = local write "Measure Ch-A"(w4544) -> ()
                              n2312 = Bundle By Name(cluster=w4536, "MAX Vpp"=w4525, "PickToPick / 2"=w4530, "MIN Vpp"=w4524) -> (w4537:T9)
                              n2313 = local write "Measure Ch-B"(w4537) -> ()
                            }
                            frame #2 {
                              # "GoTo Test-nmb"
                              # "ReTest Cyckles"
                              # "Select Channel & Set Retest Parametrs in FALSE Case"
                              n2314 = case shown="\"B\"" w4561 {
                                tunnel: [w4581 w4583] -> w4567
                                tunnel: w4566 -> [w4581 _]
                                tunnel: [w4580 w4582] -> w4565
                                tunnel: w4564 -> [w4580 _]
                                tunnel: w4563 -> [_ w4583]
                                tunnel: w4562 -> [_ w4582]
                                frame "A", Default {
                                }
                                frame "B" {
                                }
                              }
                              n2315 = Index Array(array=w4554, index #1=0 ("index"), index #2=1 ("index"), index #3=2 ("index")) -> (element #1=w4558:string, element #2=w4559:string, element #3=w4560:string)
                              n2316 = global read "Global Variable.vi" "Retest Cnt"() -> (w4553:i16)
                              n2317 = local read "Debugging"() -> (w4551:bool)
                              n2318 = To Upper Case(1:w4558) -> (0:w4550:string)
                              n2319 = Decimal String To Number(string=w4560) -> (number=w4547:i32)  [unwired: 2 in, 1 out]
                              n2320 = Decimal String To Number(string=w4559) -> (number=w4549:i32)  [unwired: 2 in, 1 out]
                              n2321 = Equal?(x=w4553, y=i16 0) -> (x = y?=w4548:bool)
                              n2322 = case shown="False" w4551 {
                                tunnel: w4550 -> [w4571 _]
                                tunnel: w4548 -> [w4568 _]
                                tunnel: w4547 -> [w4570 _]
                                tunnel: w4549 -> [w4569 _]
                                frame False {
                                n2323 = case shown="\"FALSE\"" w4571 {
                                tunnel: w4568 -> [_ w4575]
                                tunnel: w4570 -> [_ w4572]
                                tunnel: w4569 -> [_ w4573]
                                frame "Idle", Default {
                                }
                                frame "FALSE" {
                                n2324 = global write "Global Variable.vi" "Retest Step Nmb"(w4573) -> ()
                                n2325 = global write "Global Variable.vi" "Retest Nmb"(w4572) -> ()
                                n2326 = case shown="True" w4575 {
                                tunnel: w4572 -> [_ w4579]
                                tunnel: w4573 -> [_ _]
                                frame False {
                                n2327 = global read "Global Variable.vi" "Retest Cnt"() -> (w4577:i16)
                                n2328 = Decrement(x=w4577) -> (x-1=w4576:i16)
                                n2329 = global write "Global Variable.vi" "Retest Cnt"(w4576) -> ()
                                }
                                frame True {
                                # "if(Retest-OFF & Cnt=0)"
                                n2330 = Decrement(x=w4579) -> (x-1=w4578:i32)
                                n2331 = global write "Global Variable.vi" "Retest Cnt"(w4578) -> ()
                                }
                                }
                                n2332 = global write "Global Variable.vi" "Retest ON"(TRUE ("Retest ON")) -> ()
                                }
                                }
                                }
                                frame True {
                                }
                              }
                            }
                          }
                          n2333 = in-place {
                            in-place-border: w4452 -> [_]
                            in-place-border: w4453 -> [w4476]
                            in-place-border: w4454 -> [w4474]
                            in-place-border: w4455 -> [w4473]
                            in-place-border: [w4479] -> w4466
                            in-place-border: [w4478] -> w4465
                            # "Step Result Msg"
                            # "Step TEST Result"
                            n2334 = In Range and Coerce(upper limit=w4474, x=w4476, lower limit=w4473) -> (In Range?=w4475:bool)  [unwired: 1 out]
                            n2335 = case shown="False" w4475 {
                              tunnel: [enum16{"Idle", "PASS", "FALSE"}."FALSE" ("Step Test Result") enum16{"Idle", "PASS", "FALSE"}."PASS" ("Step Test Result")] -> w4479
                              frame False {
                              }
                              frame True {
                              }
                            }
                            n2336 = Format Into String(format string="%.1f (VAC)", w4476) -> (resulting string=w4478:string)  [unwired: 2 in, 1 out]
                          }
                        }
                        frame 55 {
                          # "PicoScope\n     Case\nLower Limit"
                          # "Read Arrays Of DATA"
                          # "PicoScope AWG"
                          n2337 = Unbundle By Name(w4601) -> ("Parameters"=w4595:string, "Test Values.Upper Limit"=w4599:dbl, "Test Values.Lower Limit"=w4598:dbl, "Test Values.Numeric Value"=w4600:dbl)
                          n2338 = property on="Tab Control Msg" class="TabCtl (strict)"("Value"=T21."Settings" ("Tab Control Msg")) -> (error out=w4597:errorcluster)  [unwired: 2 in, 1 out]
                          n2339 = flat-sequence {
                            tunnel: w4600 -> [w4625]
                            tunnel: w4599 -> [w4618]
                            tunnel: w4598 -> [w4617]
                            tunnel: w4597 -> [_]
                            tunnel: [w4618] -> _
                            tunnel: [w4617] -> _
                            tunnel: w4595 -> [w4616]
                            tunnel: [w4614] -> w4594
                            tunnel: [w4608] -> w4591
                            tunnel: [w4607] -> w4590
                            tunnel: [w4606] -> w4589
                            tunnel: [w4605] -> w4588
                            tunnel: [w4604] -> w4587
                            tunnel: w4594 -> [w4653]
                            tunnel: w4591 -> [w4652]
                            tunnel: w4590 -> [w4651]
                            tunnel: w4589 -> [w4650]
                            tunnel: w4588 -> [w4649]
                            tunnel: w4587 -> [w4648]
                            tunnel: [w4635] -> w4586
                            frame #0 {
                              n2340 = while {
                                shift-right: [w4632] -> _
                                shift-left: w4616 -> [w4633]
                                tunnel: [w4628] -> w4615 mode=indexing
                                tunnel: [w4627] -> w4604
                                i -> [w4627]
                                stop <- w4631 stop-if-true
                                # "Get Array of Parametrs"
                                n2341 = Match Pattern(string=w4633, regular expression=">") -> (before substring=w4629:string, after substring=w4632:string, offset past match=w4630:i32)  [unwired: 1 in, 1 out]
                                n2342 = Less Than 0?(x=w4630) -> (x < 0?=w4631:bool)
